vi "Helper SubVI - Cepstrum Liftering.vi"(7 "lift range":i32, 10 "base t":dbl[](array[numeric]), 11 "cepstrum in":cluster{"t0":dbl, "dt":dbl, "Cx":dbl[]} {"Cx" format="%.2f"; "dt" format="%.2f"; "t0" format="%.2f"}) -> (0 "error":i32, 2 "liftering mask":cluster{"t0":dbl, "dt":dbl, "Cx":dbl[]} {"Cx" format="%.2f"; "dt" format="%.2f"; "t0" format="%.2f"}, 3 "cepstrum out":cluster{"t0":dbl, "dt":dbl, "Cx":dbl[]} {"Cx" format="%.2f"; "dt" format="%.2f"; "t0" format="%.2f"})   [LabVIEW 2023]
doc: "Sets the peaks in a cepstrum to zero."
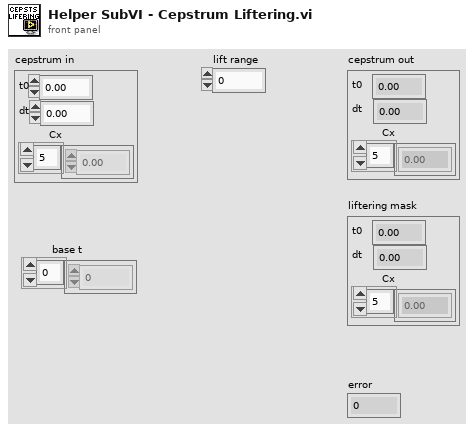
[diagram p1: front panel]
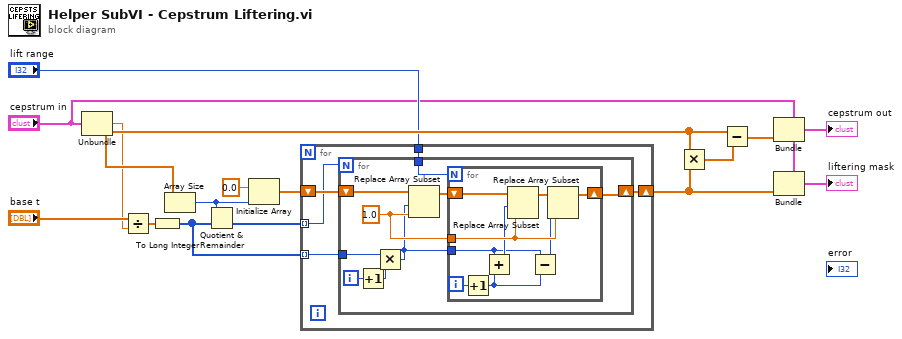
[diagram p0: block diagram]
diagram:
  n1 = Unbundle("cepstrum in") -> ("dt"=w7:dbl, "Cx"=w11:dbl[])  [unwired: 1 out]
  n2 = Divide(x="base t", y=w7) -> (x/y=w6:dbl[])
  n3 = To Long Integer(number=w6) -> (32bit integer=w5:i32[])
  n4 = Array Size(array=w11) -> (size(s)=w15:i32)
  n5 = Quotient & Remainder(x=w15, y=w5) -> (floor(x/y)=w13:i32[])  [unwired: 1 out]
  n6 = Initialize Array(0.0 ("element"), w15) -> (w14:dbl[])
  n7 = for {
    tunnel: w13 -> [w20] mode=indexing
    shift-right: [w18] -> w2
    shift-left: w14 -> [w21]
    tunnel: w5 -> [w19] mode=indexing
    tunnel: "lift range" -> [w17]
    n8 = for {
      N: w20 -> [_]
      shift-right: [w26] -> w18
      shift-left: w21 -> [w28]
      tunnel: w19 -> [w29]
      tunnel: w17 -> [w22]
      i -> [w30]
      w25 = 1.0 ("new element/subarray")
      n9 = Increment(x=w30) -> (x+1=w27:i32)
      n10 = Multiply(x=w29, y=w27) -> (x*y=w23:i32)
      n11 = Replace Array Subset(array=w28, new element=w25, index=w23) -> (w24:dbl[])
      n12 = for {
        N: w22 -> [_]
        tunnel: w25 -> [w36]
        shift-right: [w37] -> w26
        shift-left: w24 -> [w39]
        tunnel: w23 -> [w34]
        i -> [w33]
        n13 = Increment(x=w33) -> (x+1=w31:i32)
        n14 = Add(x=w34, y=w31) -> (x+y=w35:i32)
        n15 = Replace Array Subset(array=w39, new element=w36, index=w35) -> (w38:dbl[])
        n16 = Subtract(x=w34, y=w31) -> (x-y=w32:i32)
        n17 = Replace Array Subset(array=w38, new element=w36, index=w32) -> (w37:dbl[])
      }
    }
  }
  n18 = Multiply(x=w11, y=w2) -> (x*y=w1:dbl[])
  n19 = Subtract(x=w11, y=w1) -> (x-y=w10:dbl[])
  n20 = Bundle(cluster="cepstrum in", "Cx"=w10) -> (→"cepstrum out":cluster{"t0":dbl, "dt":dbl, "Cx":dbl[]})  [unwired: 2 out]
  n21 = Bundle(cluster="cepstrum in", "Cx"=w2) -> (→"liftering mask":cluster{"t0":dbl, "dt":dbl, "Cx":dbl[]})  [unwired: 2 out]
